vi "Mouse Simulation.vi"   [LabVIEW 2020]
uses:
  User32.dll
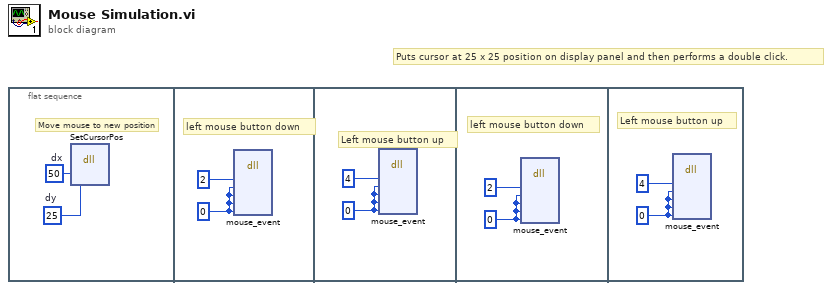
[diagram p0: block diagram]
diagram:
  # "Puts cursor at 25 x 25 position on display panel and then performs a double click."
  n1 = flat-sequence {
    frame #0 {
      w2 = 25  # dy
      w1 = 50  # dx
      # "Move mouse to new position"
      n2 = dll-call lib="User32.dll" fn="SetCursorPos" label="Move mouse to new pos"("dx"=w1, "dy"=w2) -> ()  [unwired: 6 in, 2 out]
    }
    frame #1 {
      w4 = u32 0 ("dy")
      # "left mouse button down"
      n3 = dll-call lib="user32.dll" fn="mouse_event"("dwFlags"=u32 2, "dx"=w4, "dy"=w4, "dwData"=w4, "dwExtraInfo"=w4) -> ()  [unwired: 9 in, 2 out]
    }
    frame #2 {
      w6 = u32 0 ("dy")
      # "Left mouse button up"
      n4 = dll-call lib="user32.dll" fn="mouse_event"("dwFlags"=u32 4, "dx"=w6, "dy"=w6, "dwData"=w6, "dwExtraInfo"=w6) -> ()  [unwired: 9 in, 2 out]
    }
    frame #3 {
      w7 = u32 0 ("dy")
      # "left mouse button down"
      n5 = dll-call lib="user32.dll" fn="mouse_event"("dwFlags"=u32 2, "dx"=w7, "dy"=w7, "dwData"=w7, "dwExtraInfo"=w7) -> ()  [unwired: 9 in, 2 out]
    }
    frame #4 {
      w9 = u32 0 ("dy")
      # "Left mouse button up"
      n6 = dll-call lib="user32.dll" fn="mouse_event"("dwFlags"=u32 4, "dx"=w9, "dy"=w9, "dwData"=w9, "dwExtraInfo"=w9) -> ()  [unwired: 9 in, 2 out]
    }
  }
